vi "NIIE_Template_MouseDown.vi"(7 "Add To Undo?":bool=TRUE, 8 "Error":errorcluster, 10 "CtlRef":refnum<vi>, 11 "Data":T1={"Class"={"Ants"=refnum, "Layer"=refnum, "Templates"=refnum, "Icon"=refnum, "Glyph"=refnum, "Settings"=refnum, "Tools"=refnum}, "Ref"={"Add Layer"=refnum, "Remove Layer"=refnum, "Line Text"=[], "Body Text Spec"=refnum, "DNL_Font"=refnum, "glyph path str"=refnum, "templates path str"=refnum, "Arrow Up"=refnum, "Arrow Down"=refnum, "IE VI Ref"=refnum, "Glyphs tree"=refnum, "Templates tree"=refnum, "Layer Icon Text"=refnum, "Layer Template"=refnum, "Clipboard"=refnum, "BW icon in"=refnum, "Color icon in"=refnum, "Layer Clust"=refnum, "Body Text"=refnum, "DNL_Framework Templates"=refnum, "Search Templates"=refnum, "TextMarker"=refnum, "Tab Control"=refnum, "Search Glyphs"=refnum, "Line Color"=refnum, "DNL_Glyphs []"=refnum, "Fill Color"=refnum, "Tools"=refnum, "Glyphs tree"=refnum, "Icon"=refnum, "Preview"=refnum, "Ants"=refnum, "Terminals"=refnum, "menu reference"=refnum, "LayerNames"=[], "GlyphLoadAnimation"=refnum, "TemplateLoadAnimation"=refnum, "refreshGlyphs"=refnum, "refreshTemplates"=refnum}, "Support"={"AntsRect"={"left"=0, "top"=0, "right"=0, "bottom"=0}, "Mouse Move Coords"={"Horizontal"=0, "Vertical"=0}, "Mouse Down Coords"={"Horizontal"=0, "Vertical"=0}, "Temp Coord"={"Horizontal"=0, "Vertical"=0}, "Action"=enum."Default", "Edge Color"=4914962, "Fill Color"=16860, "Mouse Down?"=FALSE, "Draft Mode?"=FALSE, "Temp Icon"=bytes[3102], "CTRL Pressed"=FALSE, "Move Selection?"=FALSE, "AntsRect Orig"={"left"=0, "top"=0, "right"=0, "bottom"=0}, "Text"="", "TM Set?"=FALSE, "Mouse inside icon?"=FALSE, "Tool (old value)"=0, "Pencil Move Color"=0, "Swap Colors?"=FALSE, "Shift pressed?"=FALSE}}) -> (0 "Error Out":errorcluster, 3 "Data Out":T1={"Class"={"Ants"=refnum, "Layer"=refnum, "Templates"=refnum, "Icon"=refnum, "Glyph"=refnum, "Settings"=refnum, "Tools"=refnum}, "Ref"={"Add Layer"=refnum, "Remove Layer"=refnum, "Line Text"=[], "Body Text Spec"=refnum, "DNL_Font"=refnum, "glyph path str"=refnum, "templates path str"=refnum, "Arrow Up"=refnum, "Arrow Down"=refnum, "IE VI Ref"=refnum, "Glyphs tree"=refnum, "Templates tree"=refnum, "Layer Icon Text"=refnum, "Layer Template"=refnum, "Clipboard"=refnum, "BW icon in"=refnum, "Color icon in"=refnum, "Layer Clust"=refnum, "Body Text"=refnum, "DNL_Framework Templates"=refnum, "Search Templates"=refnum, "TextMarker"=refnum, "Tab Control"=refnum, "Search Glyphs"=refnum, "Line Color"=refnum, "DNL_Glyphs []"=refnum, "Fill Color"=refnum, "Tools"=refnum, "Glyphs tree"=refnum, "Icon"=refnum, "Preview"=refnum, "Ants"=refnum, "Terminals"=refnum, "menu reference"=refnum, "LayerNames"=[], "GlyphLoadAnimation"=refnum, "TemplateLoadAnimation"=refnum, "refreshGlyphs"=refnum, "refreshTemplates"=refnum}, "Support"={"AntsRect"={"left"=0, "top"=0, "right"=0, "bottom"=0}, "Mouse Move Coords"={"Horizontal"=0, "Vertical"=0}, "Mouse Down Coords"={"Horizontal"=0, "Vertical"=0}, "Temp Coord"={"Horizontal"=0, "Vertical"=0}, "Action"=enum."Default", "Edge Color"=4914962, "Fill Color"=16860, "Mouse Down?"=FALSE, "Draft Mode?"=FALSE, "Temp Icon"=bytes[3102], "CTRL Pressed"=FALSE, "Move Selection?"=FALSE, "AntsRect Orig"={"left"=0, "top"=0, "right"=0, "bottom"=0}, "Text"="", "TM Set?"=FALSE, "Mouse inside icon?"=FALSE, "Tool (old value)"=0, "Pencil Move Color"=0, "Swap Colors?"=FALSE, "Shift pressed?"=FALSE}})   [LabVIEW 2021]
uses:
  Controls/IE Data.ctl
  Class/Ants/Ants.lvclass
  Class/FakedArray/FakedArray.lvclass
  Class/Icon Library/Glyph.lvclass
  Class/Settings/Settings.lvclass
  Class/Tools/Tools Paint.lvclass
  vi.lib/LabVIEW Icon API/lv_icon/Classes/Icon/Icon.lvclass
  Controls/IE Classes.ctl
  Controls/References Cluster.ctl
  Controls/SupportClass.ctl
  <vilib>/Utility/miscctls.llb/LVPoint32TypeDef.ctl
  Controls/ENUM_SupportClass_Action.ctl
  vi.lib/LabVIEW Icon API/lv_icon/Controls/IEColor.ctl
  vi.lib/LabVIEW Icon API/lv_icon/Controls/LayerType.ctl
  vi.lib/LabVIEW Icon API/lv_icon/Classes/Icon Framework/Icon Framework.lvclass
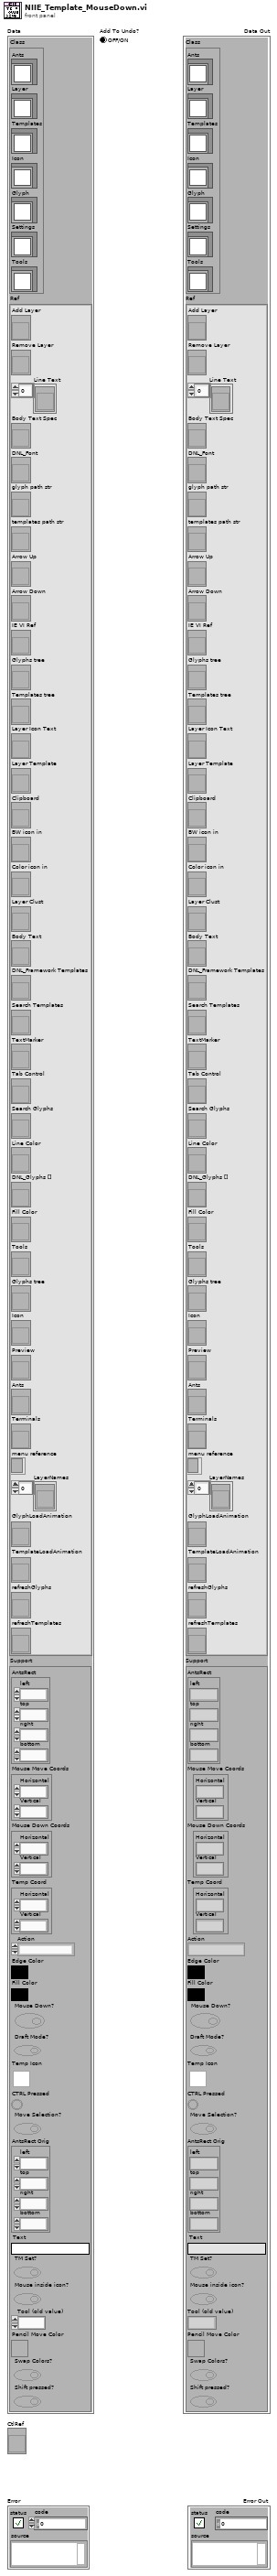
[diagram p1: front panel]
types:
  T1 = typedef "IE Data.ctl" = cluster{"Class":T2, "Ref":T3, "Support":T4}
  T2 = typedef "IE Classes.ctl" = cluster{"Ants":refnum<class "Ants.lvclass">, "Layer":refnum<class "FakedArray.lvclass">, "Templates":refnum<class "FakedArray.lvclass">, "Icon":refnum<class "Icon.lvclass">, "Glyph":refnum<class "Glyph.lvclass">, "Settings":refnum<class "Settings.lvclass">, "Tools":refnum<class "Tools Paint.lvclass">}
  T3 = typedef "References Cluster.ctl" = cluster{"Add Layer":refnum<vi>, "Remove Layer":refnum<vi>, "Line Text":refnum<vi>[], "Body Text Spec":refnum<vi>, "DNL_Font":refnum<vi>, "glyph path str":refnum<vi>, "templates path str":refnum<vi>, "Arrow Up":refnum<vi>, "Arrow Down":refnum<vi>, "IE VI Ref":refnum<vi>, "Glyphs tree":refnum<vi>, "Templates tree":refnum<vi>, "Layer Icon Text":refnum<vi>, "Layer Template":refnum<vi>, "Clipboard":refnum<vi>, "BW icon in":refnum<vi>, "Color icon in":refnum<vi>, "Layer Clust":refnum<vi>, "Body Text":refnum<vi>, "DNL_Framework Templates":refnum<vi>, "Search Templates":refnum<vi>, "TextMarker":refnum<vi>, "Tab Control":refnum<vi>, "Search Glyphs":refnum<vi>, "Line Color":refnum<vi>, "DNL_Glyphs []":refnum<vi>, "Fill Color":refnum<vi>, "Tools":refnum<vi>, "Glyphs tree":refnum<vi>, "Icon":refnum<vi>, "Preview":refnum<vi>, "Ants":refnum<vi>, "Terminals":refnum<vi>, "menu reference":refnum<k9>, "LayerNames":refnum<vi>[], "GlyphLoadAnimation":refnum<vi>, "TemplateLoadAnimation":refnum<vi>, "refreshGlyphs":refnum<vi>, "refreshTemplates":refnum<vi>}
  T4 = typedef "SupportClass.ctl" = cluster{"AntsRect":cluster{"left":i16, "top":i16, "right":i16, "bottom":i16}, "Mouse Move Coords":T5, "Mouse Down Coords":T5, "Temp Coord":T5, "Action":T6, "Edge Color":T7, "Fill Color":T7, "Mouse Down?":bool, "Draft Mode?":bool, "Temp Icon":picture, "CTRL Pressed":bool, "Move Selection?":bool, "AntsRect Orig":cluster{"left":i16, "top":i16, "right":i16, "bottom":i16}, "Text":string, "TM Set?":bool, "Mouse inside icon?":bool, "Tool (old value)":u32, "Pencil Move Color":u32, "Swap Colors?":bool, "Shift pressed?":bool}
  T5 = typedef "LVPoint32TypeDef.ctl" = cluster{"Horizontal":i32, "Vertical":i32}
  T6 = typedef "ENUM_SupportClass_Action.ctl" = enum16{"Default", "Move Selection", "Glyph Library", "Tool"}
  T7 = typedef "IEColor.ctl" = u32
  T8 = typedef "LayerType.ctl" = enum16{"Graphic", "Text", "Tool", "Graphic Drop"}
  T9 = typedef "Cluster_Path&Icon.ctl" = cluster{"Rectangle":cluster{"left":i16, "top":i16, "right":i16, "bottom":i16}, "Path":path, "Image":picture, "Filter":string, "FileName":string}
  T10 = typedef "Cluster_Layer Data.ctl" = cluster{"LayerIcon":picture, "LayerName":string, "Opacity":u8, "Visibility?":bool}
  T11 = typedef "Font.ctl" = string
  T12 = typedef "Alignment.ctl" = u16
  T13 = typedef "Font Size.ctl" = u8
  T14 = cluster{"Line 1 text":string, "Line 2 text":string, "Line 3 text":string, "Line 4 text":string, "Line 1 color":u32, "Line 2 color":u32, "Line 3 color":u32, "Line 4 color":u32, "Body Text Spec":cluster{"DNL_Font":T11, "Alignment":T12, "Size":T13}, "Center text vertically":bool, "Capitalize Text":bool}
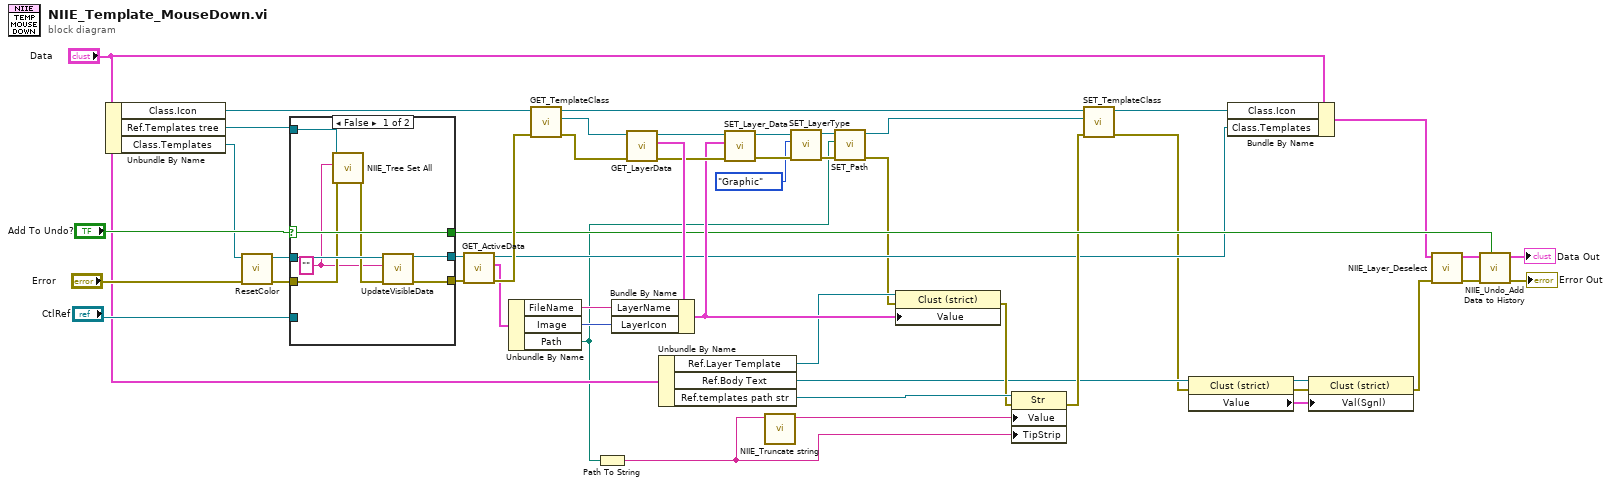
[diagram p0: block diagram]
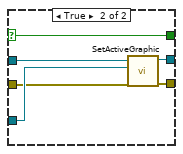
[diagram p2: hidden frame]
diagram:
  n1 = Unbundle By Name("Data") -> ("Class.Icon"=w17:refnum<class "Icon.lvclass">, "Ref.Templates tree"=w6:refnum<vi>, "Class.Templates"=w15:refnum<class "FakedArray.lvclass">)
  n2 = call "ResetColor.vi"("error in (no error)"="Error", "FakedArray in"=w15) -> ("error out"=w35:errorcluster, "FakedArray out"=w36:refnum<class "FakedArray.lvclass">)  [unwired: 8 out]
  n3 = case shown="False" "Add To Undo?" {
    selector: "Add To Undo?" -> [w57 w59]
    tunnel: "CtlRef" -> [_ w64]
    tunnel: [w56 w63] -> w49
    tunnel: [w58 w62] -> w48
    tunnel: w36 -> [w55 w61]
    tunnel: w35 -> [w52 w60]
    tunnel: [w57 w59] -> w28
    tunnel: w6 -> [w54 _]
    frame False {
      w51 = "" ("Keyword")
      n4 = call "NIIE_Tree Set All.vi"("Error"=w52, "Value"=w51, "TreeControl"=w54) -> ("Error Out"=w53:errorcluster)  [unwired: 7 in, 1 out]
      n5 = call-dynamic "UpdateVisibleData.vi"("Error"=w53, "Keyword"=w51, "FakedArray"=w55) -> ("Error Out"=w58:errorcluster, "FakedArray Out"=w56:refnum<class "FakedArray.lvclass">)  [unwired: 2 in, 5 out]
    }
    frame True {
      n6 = call-dynamic "SetActiveGraphic.vi"("error in (no error)"=w60, "Ctl Refnum"=w64, "FakedArray in"=w61) -> ("error out"=w62:errorcluster, "FakedArray out"=w63:refnum<class "FakedArray.lvclass">)  [unwired: 3 in, 4 out]
    }
  }
  n7 = call-dynamic "GET_ActiveData.vi"("Error"=w48, "FakedArray"=w49) -> ("Error Out"=w39:errorcluster, "Path And Icon Out"=w32:T9, "FakedArray Out"=w14:refnum<class "FakedArray.lvclass">)  [unwired: 7 out]
  n8 = Unbundle By Name(w32) -> ("FileName"=w23:string, "Image"=w47:picture, "Path"=w1:path)
  n9 = call-dynamic "GET_TemplateClass.vi"("error in (no error)"=w39, "Icon.lvclass in"=w17) -> ("error out"=w34:errorcluster, "Icon Framework.lvclass"=w37:refnum<class "Icon Framework.lvclass">, "Icon.lvclass out"=w40:refnum<class "Icon.lvclass">)  [unwired: 7 out]
  n10 = Path To String(path=w1) -> (string=w22:string)
  n11 = call-dynamic "GET_LayerData.vi"("error in (no error)"=w34, "Layer.lvclass in"=w37) -> ("error out"=w41:errorcluster, "Data"=w42:T10, "Layer.lvclass out"=w43:refnum<class "Icon Framework.lvclass">)  [unwired: 7 out]
  n12 = Bundle By Name(cluster=w42, "LayerName"=w23, "LayerIcon"=w47) -> (w38:T10)
  n13 = Unbundle By Name("Data") -> ("Ref.Layer Template"=w33:refnum<vi>, "Ref.Body Text"=w21:refnum<vi>, "Ref.templates path str"=w27:refnum<vi>)
  n14 = call-dynamic "SET_Layer_Data.vi"("error in (no error)"=w41, "Data"=w38, "Layer.lvclass in"=w43) -> ("error out"=w46:errorcluster, "Layer.lvclass out"=w44:refnum<class "Icon Framework.lvclass">)  [unwired: 1 in, 6 out]
  n15 = call "NIIE_Truncate string.vi"("String Path in"=w22) -> ("String path out"=w24:string)  [unwired: 1 in, 9 out]
  n16 = call-dynamic "SET_LayerType.vi"("error in (no error)"=w46, "Type"=LayerType."Graphic", "Layer.lvclass in"=w44) -> ("error out"=w3:errorcluster, "Layer.lvclass out"=w5:refnum<class "Icon Framework.lvclass">)  [unwired: 7 out]
  n17 = call "SET_Path.vi"("error in (no error)"=w3, "Path"=w1, "Icon Framework.lvclass in"=w5) -> ("error out"=w2:errorcluster, "Icon Framework.lvclass out"=w4:refnum<class "Icon Framework.lvclass">)  [unwired: 7 in]
  n18 = property class="Clust (strict)"(reference=w33, error in=w2, "Value"=w38) -> (error out=w26:errorcluster)  [unwired: 1 out]
  n19 = property class="Str"(reference=w27, error in=w26, "Value"=w24, "TipStrip"=w22) -> (error out=w25:errorcluster)  [unwired: 1 out]
  n20 = call-dynamic "SET_TemplateClass.vi"("error in (no error)"=w25, "Icon Framework.lvclass"=w4, "Icon.lvclass in"=w40) -> ("error out"=w13:errorcluster, "Icon.lvclass out"=w16:refnum<class "Icon.lvclass">)  [unwired: 7 out]
  n21 = property class="Clust (strict)"(reference=w21, error in=w13) -> (reference out=w20:refnum<vi>, error out=w19:errorcluster, "Value"=w18:T14)
  n22 = Bundle By Name(cluster="Data", "Class.Icon"=w16, "Class.Templates"=w14) -> (w11:T1)
  n23 = property class="Clust (strict)"(reference=w20, error in=w19, "Val(Sgnl)"=w18) -> (error out=w12:errorcluster)  [unwired: 1 out]
  n24 = call "NIIE_Layer_Deselect.vi"("Error"=w12, "Data"=w11) -> ("Error Out"=w31:errorcluster, "Data Out"=w10:T1)  [unwired: 8 out]
  n25 = call "NIIE_Undo_Add Data to History.vi"("Add To Undo?"=w28, "Error"=w31, "Data"=w10) -> ("Error Out"=→"Error Out":errorcluster, "Data Out"=→"Data Out":T1)  [unwired: 7 out]
